vi "Parse Starting Nodes.vi"(11 "Input":string) -> (3 "Array":string[](array[string]))   [LabVIEW 2020]
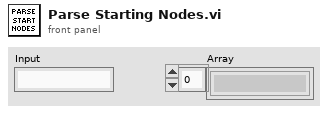
[diagram p1: front panel]
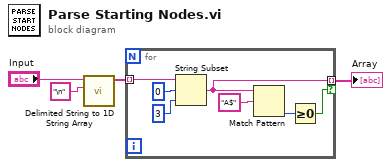
[diagram p0: block diagram]
diagram:
  n1 = call <vilib>:"Delimited String to 1D String Array.vi"("delimiter"="\n" ("search string/char (-)"), "delimited string"="Input") -> ("string array"=w2:string[])  [unwired: 9 in]
  n2 = for {
    tunnel: w2 -> [w6] mode=indexing
    tunnel: [w5] -> w4 mode=indexing if=w9
    n3 = String Subset(string=w6, offset (0)=0, length (rest)=3 ("length (rest)")) -> (substring=w5:string)
    n4 = Match Pattern(string=w5, regular expression="A$" ("y")) -> (offset past match=w10:i32)  [unwired: 1 in, 3 out]
    n5 = Greater Or Equal To 0?(x=w10) -> (x >= 0?=w9:bool)
  }
  "Array" <- w4
